vi "config timing source.vi"(8 "error in":errorcluster, 10 "DecideProjectFeatures in":refnum<class "TagBusConfigurablePluginDecideFeatures.lvclass">, 11 "User Project in":refnum<vi>) -> (0 "error out":errorcluster, 3 "User Project out":refnum<vi>)   [LabVIEW 2013, in "TagBusConfigurablePluginDecideFeatures.lvclass"]
uses:
  TagBusConfigurablePluginDecideFeatures.lvclass
  TagBusConfigurablePluginDecideFeatures.lvclass/TagBusConfigurablePluginDecideFeatures.ctl
  <vilib>/Utility/traverseref.llb/TRef TravTarget.ctl
  Read creates timing source.vi
  Read custom timing source_.vi
  Read fixed timing source name.vi
  <vilib>/Utility/traverseref.llb/VI Scripting - Traverse.lvlib
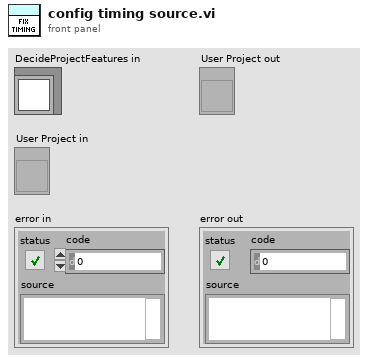
[diagram p1: front panel]
types:
  T1 = typedef "TRef TravTarget.ctl" = enum16{"FP", "BD", "Other"}
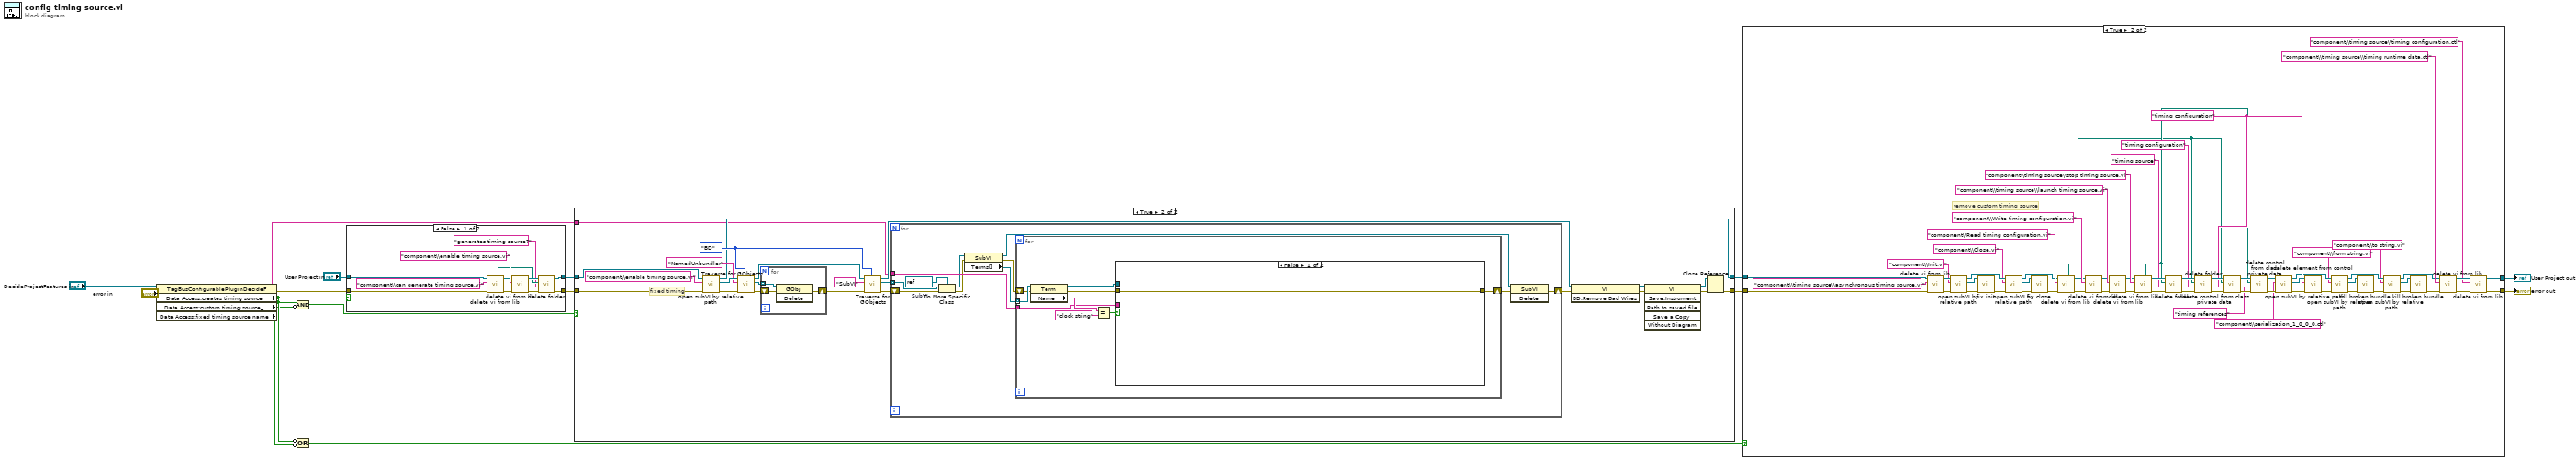
[diagram p0: block diagram]
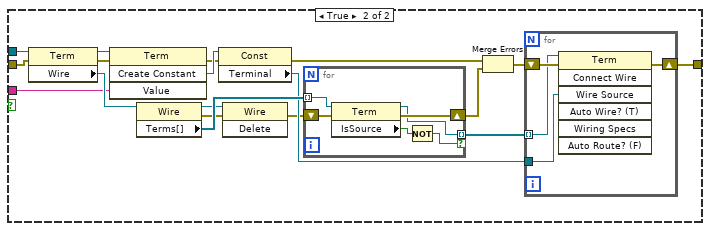
[diagram p4: hidden frame]
diagram:
  n1 = property class="TagBusConfigurablePluginDecideF"(reference="DecideProjectFeatures in", error in="error in") -> (error out=w13:errorcluster, "Data Access:creates timing source"=w11:bool, "Data Access:custom timing source_"=w10:bool, "Data Access:fixed timing source name"=w1:string)  [unwired: 1 out]
  n2 = Compound Arithmetic op=AND(w11, invert w10) -> (w9:bool)
  n3 = Compound Arithmetic op=OR(invert w11, invert w10) -> (w6:bool)
  n4 = case shown="False" w11 {
    tunnel: w13 -> [w27 w29]
    tunnel: "User Project in" -> [w26 w28]
    tunnel: [w18 w28] -> w8
    tunnel: [w19 w29] -> w7
    frame False {
      n5 = call "delete vi from lib.vi"("error in"=w27, "relative path"="component\\can generate timing source.vi", "Project in"=w26) -> ("error out"=w22:errorcluster, "Project out"=w23:refnum<vi>, "lib path"=w17:path)  [unwired: 6 in]
      n6 = call "delete vi from lib.vi"("error in"=w22, "relative path"="component\\enable timing source.vi", "Project in"=w23) -> ("error out"=w20:errorcluster, "Project out"=w21:refnum<vi>)  [unwired: 6 in, 1 out]
      n7 = call "delete folder.vi"("error in"=w20, "folder"="generates timing source?" ("relative path"), "lib path"=w17, "Project in"=w21) -> ("error out"=w19:errorcluster, "Project out"=w18:refnum<vi>)  [unwired: 6 in]
    }
    frame True {
      # "has a timing source"
    }
  }
  n8 = case shown="True" w9 {
    tunnel: w7 -> [w30 w54]
    tunnel: w8 -> [w31 w53]
    tunnel: [w31 w41] -> w4
    tunnel: [w30 w40] -> w3
    tunnel: w1 -> [_ w37]
    frame False {
    }
    frame True {
      w44 = TRef_TravTarget."BD" ("Traverse Target")
      # "fixed timing"
      n9 = call "open subVI by relative path.vi"("error in"=w54, "relative path"="component\\enable timing source.vi", "Project in"=w53) -> ("error out"=w51:errorcluster, "vi reference"=w52:refnum<vi>, "Project out"=w41:refnum<vi>)  [unwired: 6 in]
      n10 = call <vilib>:"Traverse for GObjects.vi"("Traverse Target"=w44, "error in (no error)"=w51, "Class Name"="NamedUnbundler", "VI Refnum"=w52) -> ("error out"=w48:errorcluster, "References"=w49:refnum<vi>[], "dup VI Refnum"=w46:refnum<vi>)  [unwired: 4 in, 1 out]
      n11 = for {
        tunnel: w49 -> [w105] mode=indexing
        shift-right: [w104] -> w47
        shift-left: w48 -> [w106]
        n12 = invoke class="GObj" method="Delete"(reference=w105, error in=w106) -> (error out=w104:errorcluster)  [unwired: 1 in, 2 out]
      }
      n13 = call <vilib>:"Traverse for GObjects.vi"("Traverse Target"=w44, "error in (no error)"=w47, "Class Name"="SubVI", "VI Refnum"=w46) -> ("error out"=w43:errorcluster, "References"=w33:refnum<vi>[], "dup VI Refnum"=w38:refnum<vi>)  [unwired: 4 in, 1 out]
      n14 = for {
        tunnel: w37 -> [w63]
        shift-right: [w64] -> w42
        shift-left: w43 -> [w65]
        tunnel: w33 -> [w55] mode=indexing
        w62 = refnum<vi> refnum  # SubVI
        n15 = To More Specific Class(target class=w62, reference=w55, error in=w65) -> (specific class reference=w61:refnum<vi>, error out=w60:errorcluster)
        n16 = property class="SubVI"(reference=w61, error in=w60) -> (reference out=w56:refnum<vi>, error out=w58:errorcluster, "Terms[]"=w59:refnum<vi>[])
        n17 = for {
          tunnel: w59 -> [w74] mode=indexing
          shift-right: [w68] -> w57
          shift-left: w58 -> [w73]
          tunnel: w63 -> [w66]
          n18 = property class="Term"(reference=w74, error in=w73) -> (reference out=w67:refnum<vi>, error out=w69:errorcluster, "Name"=w72:string)
          n19 = Equal?(x=w72, y="clock string" ("Class Name")) -> (x = y?=w70:bool)
          n20 = case shown="False" w70 {
            tunnel: w69 -> [w75 w93]
            tunnel: [w75 w79] -> w68
            tunnel: w67 -> [_ w92]
            tunnel: w66 -> [_ w88]
            frame False {
            }
            frame True {
              n21 = property class="Term"(reference=w92, error in=w93) -> (reference out=w91:refnum<vi>, error out=w89:errorcluster, "Wire"=w90:refnum<vi>)
              n22 = invoke class="Term" method="Create Constant"(reference=w91, error in=w89, "Value"=w88) -> (error out=w86:errorcluster, "Create Constant"=w87:refnum<vi>)  [unwired: 1 in, 2 out]
              n23 = property class="Wire"(reference=w90) -> (reference out=w76:refnum<vi>, error out=w77:errorcluster, "Terms[]"=w85:refnum<vi>[])  [unwired: 1 in]
              n24 = property class="Const"(reference=w87, error in=w86) -> (error out=w84:errorcluster, "Terminal"=w81:refnum<vi>)  [unwired: 1 out]
              n25 = invoke class="Wire" method="Delete"(reference=w76, error in=w77) -> (error out=w78:errorcluster)  [unwired: 1 in, 2 out]
              n26 = for {
                tunnel: w85 -> [w103] mode=indexing
                shift-right: [w101] -> w83
                shift-left: w78 -> [w102]
                tunnel: [w100] -> w82 mode=indexing if=w98
                n27 = property class="Term"(reference=w103, error in=w102) -> (reference out=w100:refnum<vi>, error out=w101:errorcluster, "IsSource"=w99:bool)
                n28 = Not(x=w99) -> (.not. x?=w98:bool)
              }
              n29 = Merge Errors(w84, w83) -> (w80:errorcluster)
              n30 = for {
                tunnel: w82 -> [w96] mode=indexing
                tunnel: w81 -> [w94]
                shift-right: [w95] -> w79
                shift-left: w80 -> [w97]
                n31 = invoke class="Term" method="Connect Wire"(reference=w96, error in=w97, "Wire Source"=w94) -> (error out=w95:errorcluster)  [unwired: 4 in, 6 out]
              }
            }
          }
        }
        n32 = invoke class="SubVI" method="Delete"(reference=w56, error in=w57) -> (error out=w64:errorcluster)  [unwired: 1 in, 2 out]
      }
      n33 = invoke class="VI" method="BD.Remove Bad Wires"(reference=w38, error in=w42) -> (reference out=w35:refnum<vi>, error out=w39:errorcluster)  [unwired: 1 in, 1 out]
      n34 = invoke class="VI" method="Save.Instrument"(reference=w35, error in=w39) -> (reference out=w34:refnum<vi>, error out=w36:errorcluster)  [unwired: 4 in, 4 out]
      n35 = Close Reference(reference=w34, error in (no error)=w36) -> (error out=w40:errorcluster)
    }
  }
  n36 = case shown="True" w6 {
    tunnel: [w108 w139] -> w5
    tunnel: w4 -> [w108 w124]
    tunnel: w3 -> [w107 w123]
    tunnel: [w107 w140] -> w2
    frame False {
      # "as written"
    }
    frame True {
      w144 = "timing configuration" ("Name")
      # "remove custom timing source"
      n37 = call "delete vi from lib.vi"("error in"=w123, "relative path"="component\\timing source\\asynchronous timing source.vi", "Project in"=w124) -> ("error out"=w117:errorcluster, "Project out"=w118:refnum<vi>)  [unwired: 6 in, 1 out]
      n38 = call "open subVI by relative path.vi"("error in"=w117, "relative path"="component\\Init.vi", "Project in"=w118) -> ("error out"=w112:errorcluster, "vi reference"=w114:refnum<vi>, "Project out"=w119:refnum<vi>)  [unwired: 6 in]
      n39 = call "fix init.vi"("error in"=w112, "VI in"=w114) -> ("error out"=w113:errorcluster)  [unwired: 9 in]
      n40 = call "open subVI by relative path.vi"("error in"=w113, "relative path"="component\\Close.vi", "Project in"=w119) -> ("error out"=w110:errorcluster, "vi reference"=w109:refnum<vi>, "Project out"=w120:refnum<vi>)  [unwired: 6 in]
      n41 = call "fix close.vi"("error in"=w110, "VI in"=w109) -> ("error out"=w111:errorcluster)  [unwired: 9 in]
      n42 = call "delete vi from lib.vi"("error in"=w111, "relative path"="component\\Read timing configuration.vi", "Project in"=w120) -> ("error out"=w167:errorcluster, "Project out"=w168:refnum<vi>, "lib path"=w137:path)  [unwired: 6 in]
      n43 = call "delete vi from lib.vi"("error in"=w167, "relative path"="component\\Write timing configuration.vi", "Project in"=w168) -> ("error out"=w122:errorcluster, "Project out"=w121:refnum<vi>)  [unwired: 6 in, 1 out]
      n44 = call "delete vi from lib.vi"("error in"=w122, "relative path"="component\\timing source\\launch timing source.vi", "Project in"=w121) -> ("error out"=w162:errorcluster, "Project out"=w163:refnum<vi>)  [unwired: 6 in, 1 out]
      n45 = call "delete vi from lib.vi"("error in"=w162, "relative path"="component\\timing source\\stop timing source.vi", "Project in"=w163) -> ("error out"=w161:errorcluster, "Project out"=w160:refnum<vi>, "lib path"=w138:path)  [unwired: 6 in]
      n46 = call "delete folder.vi"("error in"=w161, "folder"="timing source" ("Name"), "lib path"=w138, "Project in"=w160) -> ("error out"=w157:errorcluster, "Project out"=w158:refnum<vi>)  [unwired: 6 in]
      n47 = call "delete folder.vi"("error in"=w157, "folder"="timing configuration" ("Name"), "lib path"=w137, "Project in"=w158) -> ("error out"=w155:errorcluster, "Project out"=w154:refnum<vi>)  [unwired: 6 in]
      n48 = call "delete control from class private data.vi"("error in"=w155, "control label"=w144, "path"=w137, "Project in"=w154) -> ("error out"=w152:errorcluster, "Project out"=w153:refnum<vi>)  [unwired: 6 in]
      n49 = call "delete control from class private data.vi"("error in"=w152, "control label"="timing references", "path"=w138, "Project in"=w153) -> ("error out"=w146:errorcluster, "Project out"=w148:refnum<vi>)  [unwired: 6 in]
      n50 = call "open subVI by relative path.vi"("error in"=w146, "relative path"="component\\serialization_1_0_0_0.ctl", "Project in"=w148) -> ("error out"=w147:errorcluster, "vi reference"=w149:refnum<vi>, "Project out"=w133:refnum<vi>)  [unwired: 6 in]
      n51 = call "delete element from control.vi"("error in"=w147, "control label"=w144, "VI in"=w149) -> ("error out"=w136:errorcluster)  [unwired: 8 in]
      n52 = call "open subVI by relative path.vi"("error in"=w136, "relative path"="component\\from string.vi", "Project in"=w133) -> ("error out"=w128:errorcluster, "vi reference"=w130:refnum<vi>, "Project out"=w134:refnum<vi>)  [unwired: 6 in]
      n53 = call "kill broken bundle.vi"("error in"=w128, "VI in"=w130) -> ("error out"=w129:errorcluster)  [unwired: 9 in]
      n54 = call "open subVI by relative path.vi"("error in"=w129, "relative path"="component\\to string.vi", "Project in"=w134) -> ("error out"=w126:errorcluster, "vi reference"=w127:refnum<vi>, "Project out"=w135:refnum<vi>)  [unwired: 6 in]
      n55 = call "kill broken bundle.vi"("error in"=w126, "VI in"=w127) -> ("error out"=w125:errorcluster)  [unwired: 9 in]
      n56 = call "delete vi from lib.vi"("error in"=w125, "relative path"="component\\timing source\\timing runtime data.ctl", "Project in"=w135) -> ("error out"=w142:errorcluster, "Project out"=w143:refnum<vi>)  [unwired: 6 in, 1 out]
      n57 = call "delete vi from lib.vi"("error in"=w142, "relative path"="component\\timing source\\timing configuration.ctl", "Project in"=w143) -> ("error out"=w140:errorcluster, "Project out"=w139:refnum<vi>)  [unwired: 6 in, 1 out]
    }
  }
  "error out" <- w2
  "User Project out" <- w5
